vi "file_pathnames.vi"(0 "Animal x":i32, 8 "Action":T4, 11 "Input \nparameters":T2={"Frame rate (ms)"=2000, "Worm strain"="N2", "Time t"=0, "State"=enum."Image acquisition", "Time elapsed"=0.0, "Max_num_runs"=100000, "#TTL"=0, "Time of start TTL"=100000, "ImSub Value"=0, "Time of last TTL"=0, "Number of Columns"=2, "Number of Rows"=2, "# AdjacentTTL"=0, "Sleep deprivation status"="", "Sleep Detection"=FALSE, "# Sleep detections"=0, "Time of first sleep detection"=0, "Time max # adjacent TTL"=0, "Image t-1"=[], "Image t"=[]} {"Number of Rows" items=["1"=1, "2"=2, "3"=3, "4"=4]; "Number of Columns" items=["1"=1, "2"=2, "3"=3, "4"=4]}) -> (3 "File-path\n-names":T3)   [LabVIEW 2011]
uses:
  Action-Init-Update-Get.ctl
  state.ctl
panel:
  in  "File-path\n-names":T3
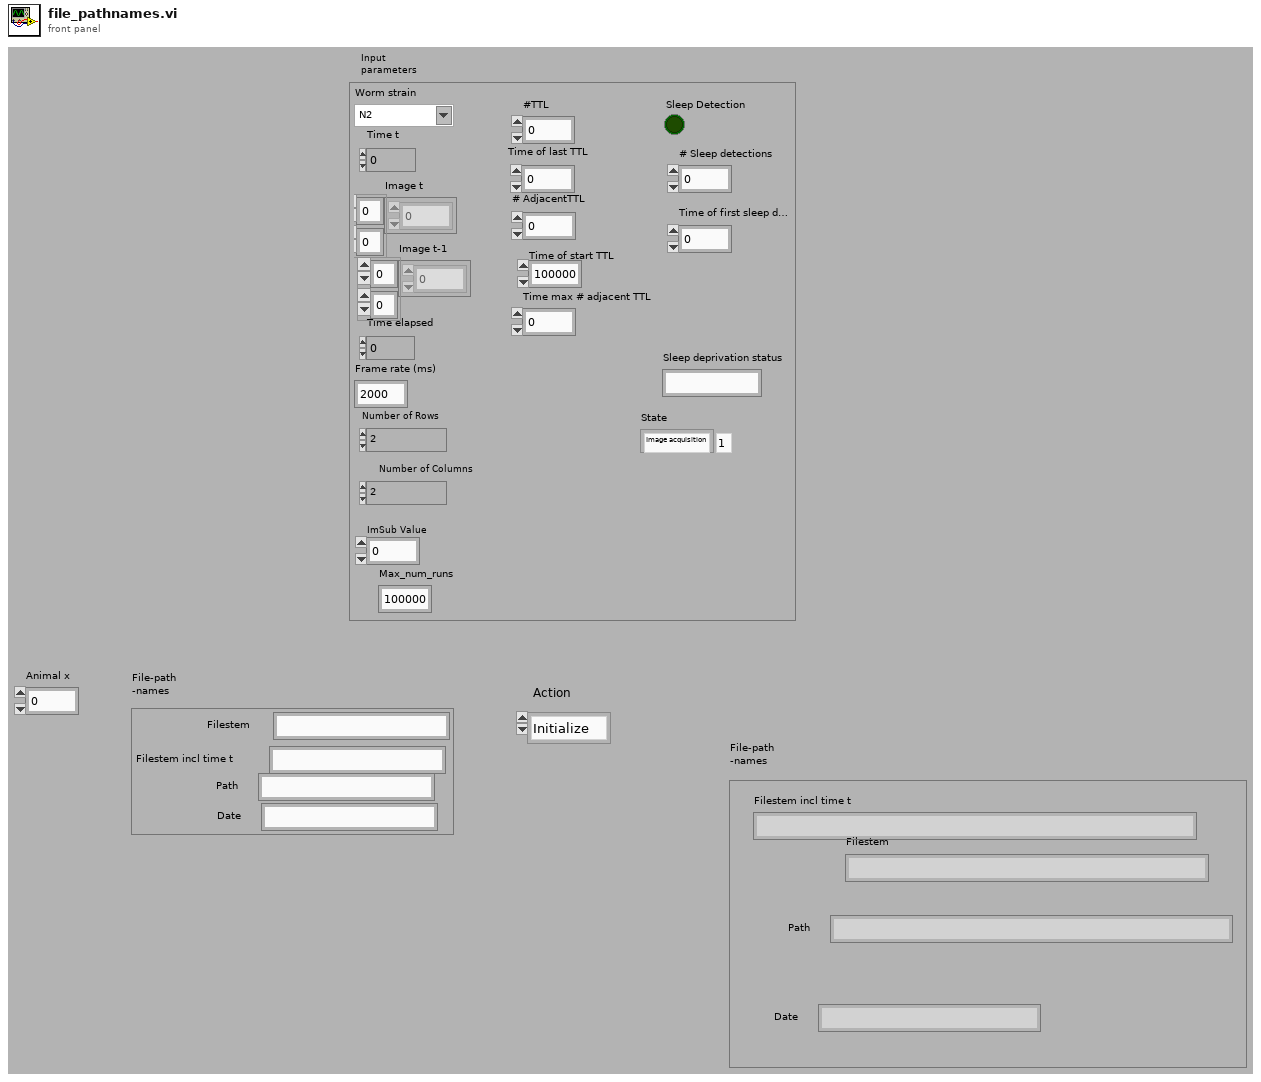
[diagram p1: front panel]
types:
  T1 = typedef "state.ctl" = enum16{"Initialize measurement", "Image acquisition", "Image processing", "Sleep detection", "Control TTL protocol ", "Sleep deprivation", "Update image & exit condition", "Wait "}
  T2 = cluster{"Frame rate (ms)":u32, "Worm strain":string, "Time t":i32, "State":T1, "Time elapsed":dbl, "Max_num_runs":i32, "#TTL":i32, "Time of start TTL":i32, "ImSub Value":i32, "Time of last TTL":i32, "Number of Columns":u32, "Number of Rows":u32, "# AdjacentTTL":i32, "Sleep deprivation status":string, "Sleep Detection":bool, "# Sleep detections":i32, "Time of first sleep detection":i32, "Time max # adjacent TTL":i32, "Image t-1":i32[][], "Image t":i32[][]}
  T3 = cluster{"Path":string, "Filestem":string, "Filestem incl time t":string, "Date":string}
  T4 = typedef "Action-Init-Update-Get.ctl" = enum16{"Initialize", "Update", "Get"}
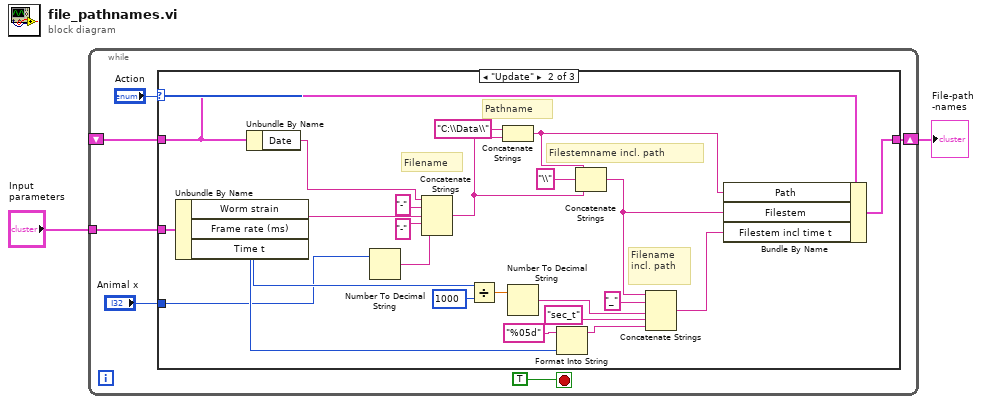
[diagram p0: block diagram]
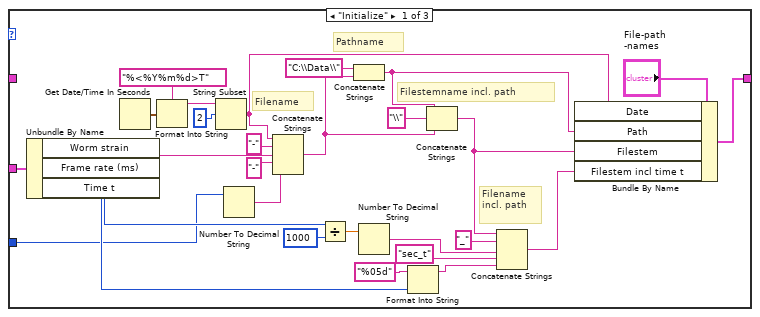
[diagram p2: hidden frame]
diagram:
  n1 = while {
    tunnel: "Input \nparameters" -> [w6]
    shift-right: [w5] -> w2
    shift-left: _ -> [w4]
    stop <- TRUE ("stop") stop-if-true
    n2 = case shown="\"Update\"" "Action" {
      tunnel: w4 -> [_ w37 w61]
      tunnel: [w30 w58 w61] -> w5
      tunnel: w6 -> [w31 w59 _]
      tunnel: "Animal x" -> [w9 w38 _]
      frame "Initialize" {
        # "Filename\nincl. path"
        # "Pathname"
        # "Filestemname incl. path"
        # "Filename"
        n3 = Unbundle By Name(w31) -> ("Worm strain"=w27:string, "Frame rate (ms)"=w15:u32, "Time t"=w14:i32)
        n4 = Get Date/Time In Seconds() -> (seconds since 1Jan1904=w35:timestamp)
        n5 = Format Into String(format string="%<%Y%m%d>T" ("Format-String"), w35) -> (resulting string=w34:string)  [unwired: 2 in, 1 out]
        n6 = String Subset(string=w34, offset (0)=2 ("Offset (0)")) -> (substring=w10:string)  [unwired: 1 in]
        n7 = Number To Decimal String(number=w9) -> (decimal integer string=w25:string)  [unwired: 1 in]
        n8 = Concatenate Strings(w10, "-" ("String"), w27, "-" ("string"), w25) -> (w23:string)
        n9 = Divide(x=w15, y=u32 1000) -> (x/y=w21:dbl)
        n10 = Concatenate Strings("C:\\Data\\", w23) -> (w11:string)
        n11 = Number To Decimal String(number=w21) -> (decimal integer string=w22:string)  [unwired: 1 in]
        n12 = Format Into String(format string="%05d" ("Format-String"), w14) -> (resulting string=w16:string)  [unwired: 2 in, 1 out]
        n13 = Concatenate Strings(w11, "\\", w23) -> (w13:string)
        n14 = Concatenate Strings(w13, "_" ("String"), w22, "sec_t" ("String"), w16) -> (w12:string)
        n15 = Bundle By Name(cluster="File-path\n-names", "Date"=w10, "Path"=w11, "Filestem"=w13, "Filestem incl time t"=w12) -> (w30:T3)
      }
      frame "Update" {
        # "Filename\nincl. path"
        # "Pathname"
        # "Filestemname incl. path"
        # "Filename"
        n16 = Unbundle By Name(w59) -> ("Worm strain"=w56:string, "Frame rate (ms)"=w44:u32, "Time t"=w43:i32)
        n17 = Unbundle By Name(w37) -> ("Date"=w39:string)
        n18 = Number To Decimal String(number=w38) -> (decimal integer string=w54:string)  [unwired: 1 in]
        n19 = Concatenate Strings(w39, "-" ("String"), w56, "-" ("string"), w54) -> (w52:string)
        n20 = Divide(x=w44, y=u32 1000) -> (x/y=w50:dbl)
        n21 = Concatenate Strings("C:\\Data\\", w52) -> (w40:string)
        n22 = Number To Decimal String(number=w50) -> (decimal integer string=w51:string)  [unwired: 1 in]
        n23 = Format Into String(format string="%05d" ("Format-String"), w43) -> (resulting string=w45:string)  [unwired: 2 in, 1 out]
        n24 = Concatenate Strings(w40, "\\", w52) -> (w42:string)
        n25 = Concatenate Strings(w42, "_" ("String"), w51, "sec_t" ("String"), w45) -> (w41:string)
        n26 = Bundle By Name(cluster=w37, "Path"=w40, "Filestem"=w42, "Filestem incl time t"=w41) -> (w58:T3)
      }
      frame "Get" {
      }
    }
  }
  "File-path\n-names" <- w2
